vi "Multi_LOG.vi"() -> ()   [LabVIEW 2014]
uses:
  <vilib>/Instr/_visa.llb/VISA Set IO Buffer Mask.ctl
  <vilib>/Instr/_visa.llb/VISA Flush IO Buffer Mask.ctl
  <vilib>/Instr/_visa.llb/VISA Configure Serial Port (Instr).vi
  picohrdl.dll
panel:
  out "Bytes":i32(graph)=253
  in  "Save?":bool=TRUE caption="Save"
  out "Nr of channels":dbl=5.0
  out "P2":dbl[](graph)=[3300.984789697503]
  out "P1":dbl[](graph)=[22.11626756552816]
  out "P5":dbl[](graph)=[616.6601916146507]
  out "P4":dbl[](graph)=[-159.04700416886857]
  out "P3":dbl[](graph)=[1339.2583006660104]
  in  "Voltage range":i32[](array[numeric])=[6, 0, 0, 0, 0, 0, 0, 0, 3, 0, 0, 0, 0, 0, 0, 0] min=0 max=6 step=1
  in  "Single ended\n(1- single)\n(0 - difer)":i32[](array[numeric])=[0, 1, 1, 1, 1, 1, 1, 1, 1, 1, 1, 1, 1, 1, 1, 1] min=0 max=1 step=1
  in  "Ch nr":bool[](array[boolean])=[TRUE, FALSE, FALSE, FALSE, TRUE, FALSE, TRUE, FALSE, TRUE, FALSE, TRUE, FALSE, FALSE, FALSE, FALSE, FALSE]
  in  "conversionTime":i16(ring)=3 items=["60 ms", "100 ms", "180 ms", "340 ms", "660 ms"]
  in  "Mains Frequency":i16(ring) items=["50 Hz", "60 Hz"]
  in  "sampleInterval_ms":i32=2500
  out "Real time":timestamp=timestamp(3598016060.195616 s since 1904-01-01)
  out "Sensor3":i32[](graph)=[0, 9682, 31275, 0, 9682, 30834, 0, 9682, 31052, 0, 9682, 31052, 0, 9682, 31057, 0, 9682, 31052, 0, 9682, 31057, 0, 9682, 30834, 0, 9682, 30839, 0, 9682, 31057, 0, 9682, 30839, 0, 9682, 30839]
  out "Sensor2":i32[](graph)=[0, 21, 96, 0, 984, 877, 0, 21, 52, 0, 19, 671, 0, 913, 467, 0, 927, 660, 0, 960, 885, 0, 982, 845, 0, 987, 396, 0, 936, 541, 0, 962, 983, 0, 975, 828]
  out "Sensor1":dbl[](graph)=[0.0, 620.021, 1359.096, 0.0, 619.984, 1358.877, 0.0, 620.021, 1359.052, 0.0, 620.019, 1358.671, 0.0, 619.913, 1358.467, 0.0, 619.927, 1358.66, 0.0, 619.96, 1357.885, 0.0, 619.982, 1357.845, 0.0, 619.987, 1357.396, 0.0, 619.936, 1358.541, 0.0, 619.962, 1357.983, 0.0, 619.975, 1357.828]
  in  "stop":bool
  in  "VISA resource name":refnum<visa-resource-name>="COM8"
  # "1       2       3      4       5        6       7       8       9      10     11      12     13    14       15     16"
  # "0 -+2500mV\n1 -+1250mV\n2 -+625mV\n3 -+313mV\n4 -+156mV\n5 -+78mv\n6 -+39mV"
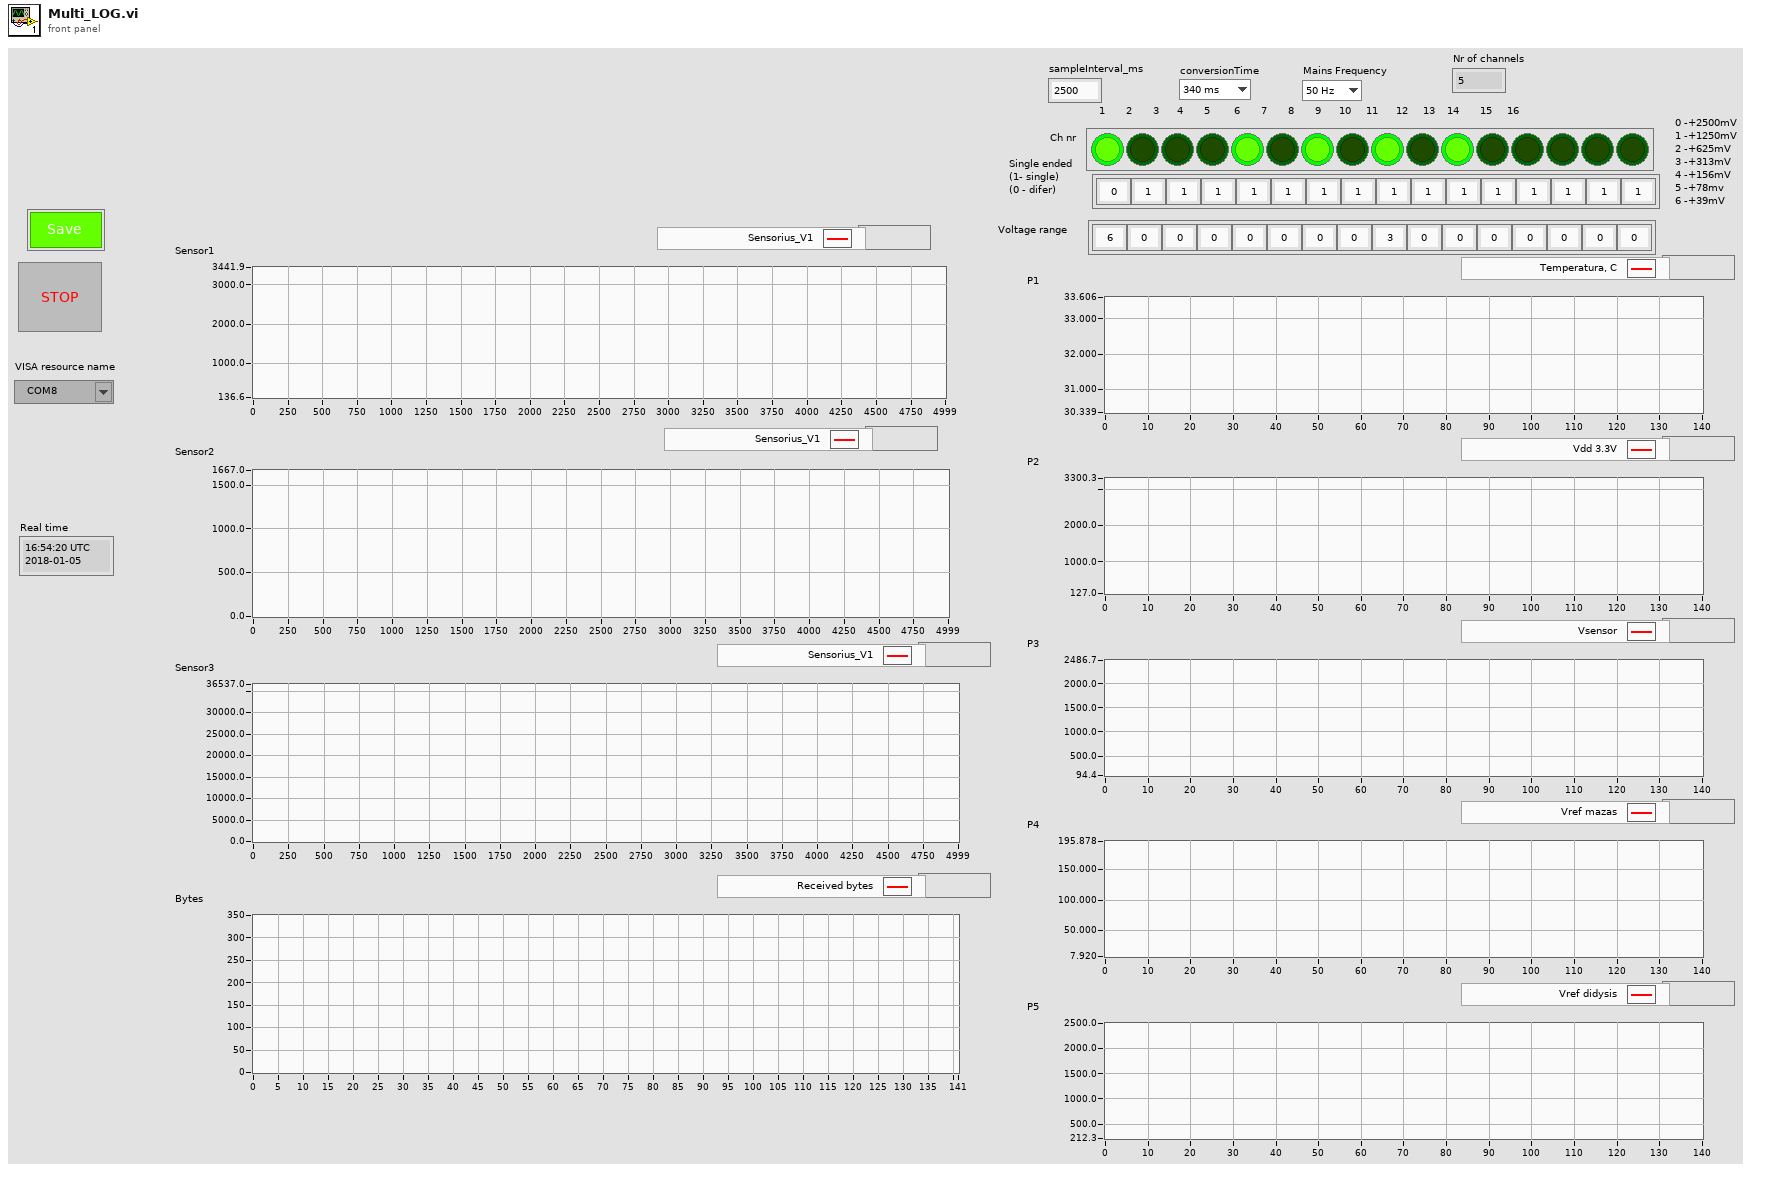
[diagram p1: front panel]
types:
  T1 = typedef "VISA Set IO Buffer Mask.ctl" = u16
  T2 = typedef "VISA Flush IO Buffer Mask.ctl" = u16
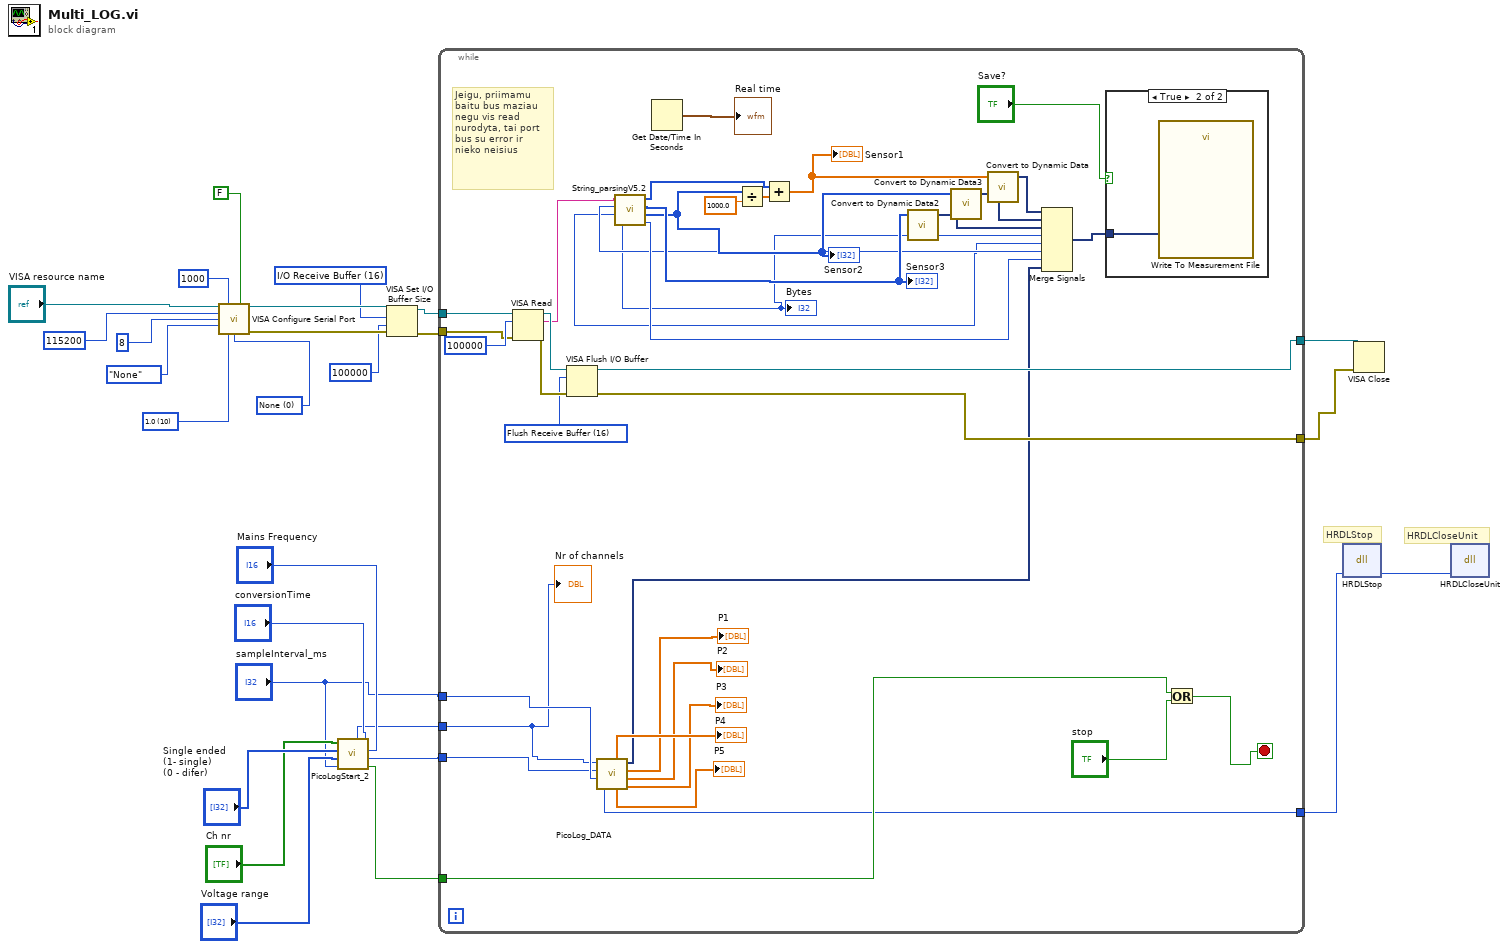
[diagram p0: block diagram]
diagram:
  w17 = T1 16 items=["I/O Receive Buffer"=16, "I/O Transmit Buffer"=32, "I/O Receive and Transmit Buffer"=48] ("Mask")
  w23 = u16 0 items=["None", "XON/XOFF", "RTS/CTS", "XON/XOFF & RTS/CTS", "DTR/DSR", "XON/XOFF & DTR/DSR"] ("flow control (0:none)")
  w24 = u16 10 items=["1.0"=10, "1.5"=15, "2.0"=20] ("stop bits (10: 1 bit)")
  # "HRDLStop"
  # "HRDLCloseUnit"
  n1 = call-poly "VISA Configure Serial Port"("VISA resource name"="VISA resource name", "timeout (10sec)"=u32 1000, "Enable Termination\nChar (T)"=FALSE ("Enable Termination\nChar (T)"), "baud rate (9600)"=u32 115200, "data bits (8)"=u16 8, "parity (0:none)"=enum16{"None", "Odd", "Even", "Mark", "Space"}."None", "stop bits (10: 1 bit)"=w24, "flow control (0:none)"=w23) -> ("VISA resource name out"=w19:refnum<visa-resource-name>, "error out"=w20:errorcluster)  [unwired: 6 in]
  n2 = call "PicoLogStart_2.vi"("Ch nr"="Ch nr", "Single ended\n(0- single)\n(1 - difer)"="Single ended\n(1- single)\n(0 - difer)", "Voltage range"="Voltage range", "sampleInterval_ms"="sampleInterval_ms", "conversionTime"="conversionTime", "Mains Frequency"="Mains Frequency") -> ("noOfChannels"=w5:i16, "handle"=w4:i16, "STOP"=w3:bool)
  n3 = VISA Set I/O Buffer Size(VISA resource name=w19, mask (16)=w17, size (4096)=u32 100000, error in (no error)=w20) -> (VISA resource name out=w14:refnum<visa-resource-name>, error out=w16:errorcluster)
  n4 = while {
    tunnel: w14 -> [w65]
    tunnel: w16 -> [w63]
    tunnel: [w59] -> w13
    tunnel: [w58] -> w12
    tunnel: "sampleInterval_ms" -> [w37]
    tunnel: w5 -> [w30]
    tunnel: w4 -> [w36]
    tunnel: w3 -> [w35]
    tunnel: [w31] -> w1
    stop <- w33 stop-if-true
    w60 = T2 16 items=["Flush Receive Buffer"=16, "Write Transmit Buffer to Device"=32, "Flush Receive Buffer (No I/O)"=64, "Flush Transmit Buffer"=128] ("Mask")
    # "Jeigu, priimamu baitu bus maziau negu vis read nurodyta, tai port bus su error ir nieko neisius"
    n5 = VISA Read(VISA resource name=w65, byte count=u32 100000, error in (no error)=w63) -> (VISA resource name out=w62:refnum<visa-resource-name>, read buffer=w49:string, error out=w61:errorcluster)  [unwired: 1 out]
    n6 = VISA Flush I/O Buffer(VISA resource name=w62, mask (16)=w60, error in (no error)=w61) -> (VISA resource name out=w59:refnum<visa-resource-name>, error out=w58:errorcluster)
    n7 = call "PicoLog_DATA.vi"("noOfChannels"=w30, "handle"=w36, "sampleInterval_ms"=w37) -> ("handle"=w31:i16, "P4"=→"P4":dbl[], "P5"=→"P5":dbl[], "Waveform Graph 3"=w32:dynamicdata, "P1"=→"P1":dbl[], "P2"=→"P2":dbl[], "P3"=→"P3":dbl[])
    n8 = call "String_parsingV5.2.vi"("input string"=w49) -> ("hour"=w48:i32, "V2"=w45:i32[], "V3"=w46:i32[], "V1"=w47:i32[], "size(s)"=w28:i32, "sekundes"=w43:i32, "minute"=w44:i32)
    "Sensor2" <- w45
    "Sensor3" <- w46
    "Bytes" <- w28
    n9 = Get Date/Time In Seconds() -> (seconds since 1Jan1904=→"Real time":timestamp)
    n10 = Divide(x=w45, y=1000.0) -> (x/y=w53:dbl[])
    n11 = Add(x=w47, y=w53) -> (x+y=w51:dbl[])
    "Sensor1" <- w51
    n12 = call "Convert to Dynamic Data2"("Array"=w46) -> ("Dynamic Data Type"=w56:dynamicdata)  [unwired: 3 in]
    n13 = call "Convert to Dynamic Data3"("Array"=w45) -> ("Dynamic Data Type"=w55:dynamicdata)  [unwired: 3 in]
    n14 = call "Convert to Dynamic Data"("Array"=w51) -> ("Dynamic Data Type"=w57:dynamicdata)  [unwired: 3 in]
    n15 = Merge Signals(w57, w55, w56, w28, w43, w44, w48, w32) -> (w50:dynamicdata)
    n16 = case shown="True" "Save?" {
      tunnel: w50 -> [_ w66]
      frame False {
      }
      frame True {
        n17 = call "Write To Measurement File"("Signals"=w66) -> ()  [unwired: 16 in, 3 out]
      }
    }
    n18 = Or(x=w35, y="stop") -> (x .or. y?=w33:bool)
    "Nr of channels" <- w30
  }
  n19 = dll-call lib="picohrdl.dll" fn="HRDLStop"("handle"=w1) -> ("handle"=w2:i16)  [unwired: 4 in, 2 out]
  n20 = VISA Close(VISA resource name=w13, error in (no error)=w12) -> ()  [unwired: 1 out]
  n21 = dll-call lib="PicoHRDL.dll" fn="HRDLCloseUnit"("handle"=w2) -> ()  [unwired: 5 in, 2 out]
